vi "ConvertPrefStrings.vi"(6 "Comma?":bool, 8 "String In":string, 11 "Settings":T1={"Name of test"="", "Date"=timestamp(0 s since 1904-01-01), "Location"="Home", "Template"="Simple", "Soundcard"="OCTA-CAPTURE", "resolution"=32, "Sampling rate"=48000, "Ch1 Gain "=25.0, "Ch2 Gain"=10.0, "Sample time (s)"=0.3, "Pre-trigger (s)"=0.001, "Hammer Threshold"=10.0, "Positions"=12, "Taps/Position"=5, "Set Names"="H,V", "Freq resolution"=1.0, "Hammer cutoff"=0.025, "Mic cutoff"=0.25, "Double bounce "=10.0, "Hammer Cal"=10.0, "dB Offset"=0.0, "Accel Cal"=10.0, "Vibrometer Cal"=0.0, "Mic Cal"=0.0, "Output"=2, "Voltage Cal"=0.01, "Vibrometer Port"="ASRL27::INSTR", "Range"=4, "High Pass"=2, "Bandwidth"=4, "X Range"=[], "Y Range"=[], "dB Spread"=0.0, "Trigger"=0, "Ch_1"=25, "Ch_2"=25, "flip?"=FALSE, "60Hz"=FALSE, "Time offset"=0.0, "Piezo Cal"=1.0, "Default Notes"=""} {"Ch_2" min=1 step=1; "Ch_1" min=1 max=100 step=1; "Trigger" items=["Hammer (force)", "Self-tap", "Spacebar"]; "Bandwidth" items=["1 kHz"=1, "5 kHz"=5, "10 kHz"=10, "25 kHz"=25, "50 kHz"=50, "100 kHz"=100]; "High Pass" items=["Off", "13 Hz", "104 Hz"]; "Range" items=["10 mm/s"=1, "20 mm/s"=2, "50 mm/s"=5, "100 mm/s"=10, "200 mm/s"=20, "500 mm/s"=50, "1 m/s"=100, "2 m/s"=200]; "Output" items=["Accelerometer", "Speed (from acceleration)", "Microphone", "Vibrometer", "Piezo"]; "Voltage Cal" format="%#_13g"; "Ch2 Gain" format="%#_13g"; "Ch1 Gain" format="%#_13g"; "Double bounce" min=0.0; "Mic cutoff" min=0.0 format="%#_4g"; "Hammer cutoff" min=0.0 format="%#_4g"; "Freq resolution" min=0.0; "Pre-trigger (s)" format="%#_13g"; "Date" format="%<%H:%M\n%d/%m/%y>T"; "resolution" items=["16 bit"=16, "24 bit"=24, "32 bit"=32]; "Sampling rate" items=["22050 samp/s"=22050, "44100 samp/s"=44100, "48000 samp/s"=48000]}) -> (0 "Settings":T1={"Name of test"="", "Date"=timestamp(0 s since 1904-01-01), "Location"="", "Template"="", "Soundcard"="", "resolution"=32, "Sampling rate"=48000, "Ch1 Gain "=25.0, "Ch2 Gain"=10.0, "Sample time (s)"=0.3, "Pre-trigger (s)"=0.01, "Hammer Threshold"=10.0, "Positions"=12, "Taps/Position"=5, "Set Names"="", "Freq resolution"=10.0, "Hammer cutoff"=0.0, "Mic cutoff"=0.0, "Double bounce "=0.0, "Hammer Cal"=10.0, "dB Offset"=0.0, "Accel Cal"=10.0, "Vibrometer Cal"=0.0, "Mic Cal"=0.0, "Output"=2, "Voltage Cal"=0.01, "Vibrometer Port"="ASRL27::INSTR", "Range"=4, "High Pass"=2, "Bandwidth"=4, "X Range"=[], "Y Range"=[], "dB Spread"=0.0, "Trigger"=0, "Ch_1"=25, "Ch_2"=25, "flip?"=FALSE, "60Hz"=FALSE, "Time offset"=0.0, "Piezo Cal"=1.0, "Default Notes"=""} {"Ch_2" min=1 step=1; "Ch_1" min=1 max=100 step=1; "Trigger" items=["Hammer (force)", "Self-tap", "Spacebar"]; "Bandwidth" items=["1 kHz"=1, "5 kHz"=5, "10 kHz"=10, "25 kHz"=25, "50 kHz"=50, "100 kHz"=100]; "High Pass" items=["Off", "13 Hz", "104 Hz"]; "Range" items=["10 mm/s"=1, "20 mm/s"=2, "50 mm/s"=5, "100 mm/s"=10, "200 mm/s"=20, "500 mm/s"=50, "1 m/s"=100, "2 m/s"=200]; "Output" items=["Accelerometer", "Speed (from acceleration)", "Microphone", "Vibrometer", "Piezo"]; "Voltage Cal" format="%#_13g"; "Ch2 Gain" format="%#_13g"; "Ch1 Gain" format="%#_13g"; "Double bounce" min=0.0; "Mic cutoff" min=0.0 format="%#_4g"; "Hammer cutoff" min=0.0 format="%#_4g"; "Freq resolution" min=0.0; "Pre-trigger (s)" format="%#_13g"; "Date" format="%<%H:%M\n%d/%m/%y>T"; "resolution" items=["16 bit"=16, "24 bit"=24, "32 bit"=32]; "Sampling rate" items=["22050 samp/s"=22050, "44100 samp/s"=44100, "48000 samp/s"=48000]}, 3 "String Out":string)   [LabVIEW 2022 SP3]
uses:
  PreferencesControl.ctl
  <vilib>/Utility/error.llb/Trim Whitespace One-Sided.vi
  Mic/Mic_Global.vi
panel:
  # "Hz"
  # "dB"
  # "dB"
  # "sec"
  # "sec"
  # "mV/Pa"
  # "mV/m/s2"
  # "mV/mm/s"
  # "V/N"
  # "sec"
  # "sec"
  # "mV/N"
  # "a.u."
  # "a.u."
  # "sec"
  # "Hz"
  # "dB"
  # "dB"
  # "sec"
  # "sec"
  # "mV/Pa"
  # "mV/m/s2"
  # "mV/mm/s"
  # "V/N"
  # "sec"
  # "sec"
  # "mV/N"
  # "a.u."
  # "a.u."
  # "sec"
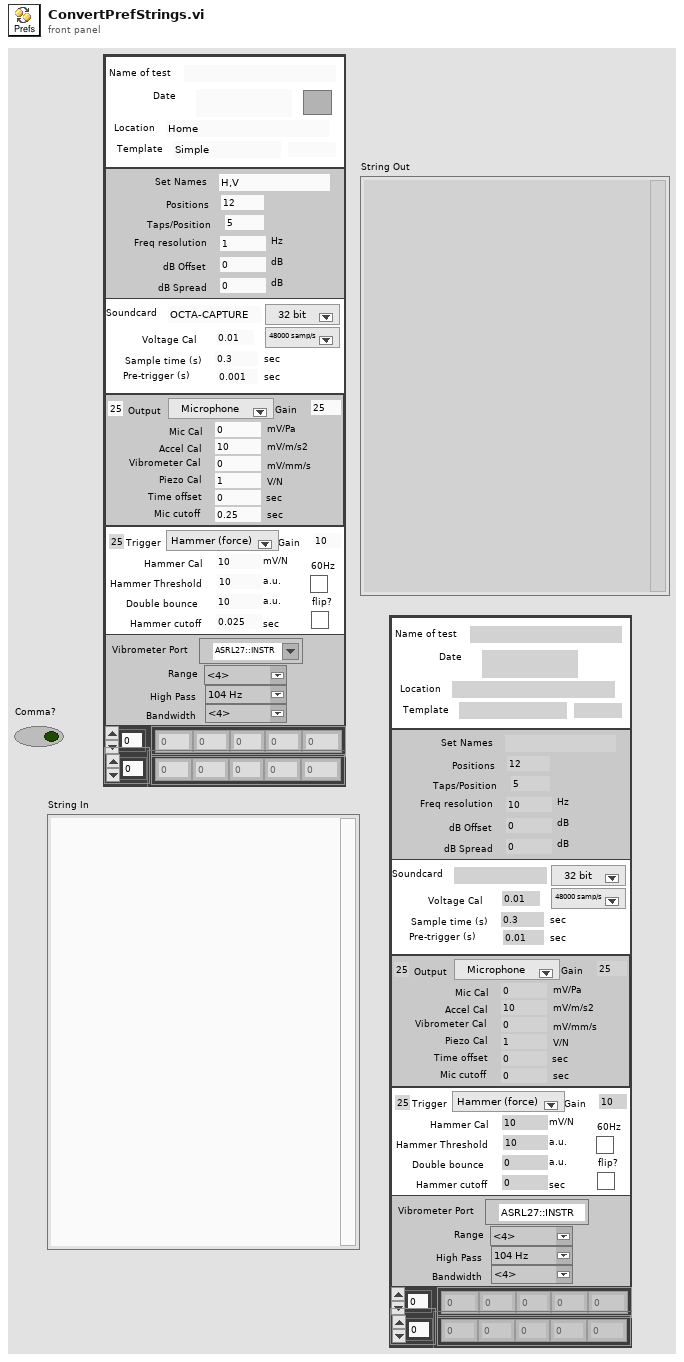
[diagram p1: front panel]
types:
  T1 = typedef "PreferencesControl.ctl" = cluster{"Name of test":string, "Date":timestamp, "Location":string, "Template":string, "Soundcard":string, "resolution":u16, "Sampling rate":u16, "Ch1 Gain ":dbl, "Ch2 Gain":dbl, "Sample time (s)":dbl, "Pre-trigger (s)":dbl, "Hammer Threshold":dbl, "Positions":i16, "Taps/Position":i16, "Set Names":string, "Freq resolution":dbl, "Hammer cutoff":dbl, "Mic cutoff":dbl, "Double bounce ":dbl, "Hammer Cal":dbl, "dB Offset":dbl, "Accel Cal":dbl, "Vibrometer Cal":dbl, "Mic Cal":dbl, "Output":u16, "Voltage Cal":dbl, "Vibrometer Port":refnum<visa-resource-name>, "Range":u16, "High Pass":u16, "Bandwidth":u16, "X Range":cluster{"Minimum":dbl, "Maximum":dbl, "Increment":dbl, "Minor Increment":dbl, "Start":dbl}[], "Y Range":cluster{"Minimum":dbl, "Maximum":dbl, "Increment":dbl, "Minor Increment":dbl, "Start":dbl}[], "dB Spread":dbl, "Trigger":u16, "Ch_1":u8, "Ch_2":u8, "flip?":bool, "60Hz":bool, "Time offset":dbl, "Piezo Cal":dbl, "Default Notes":string}
  T2 = typedef "LVStringsAndValuesArrayTypeDef_U16.ctl" = cluster{"String":string, "Value":u16}[]
  T3 = cluster{"Minimum":dbl, "Maximum":dbl, "Increment":dbl, "Minor Increment":dbl, "Start":dbl}[]
  T4 = cluster{"[0]":dbl, "[1]":dbl, "[2]":dbl, "[3]":dbl, "[4]":dbl}
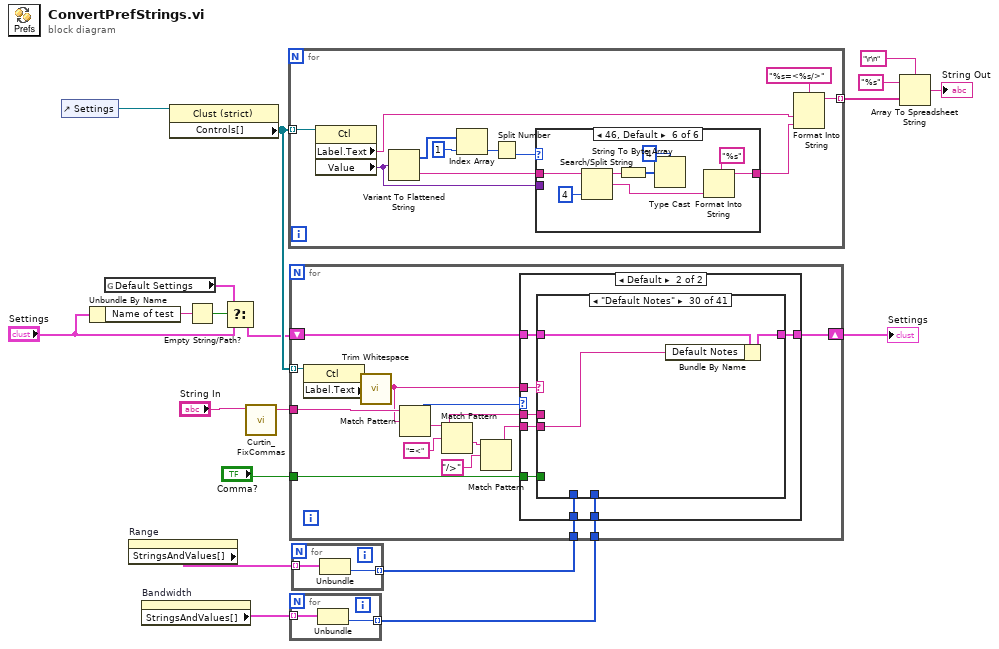
[diagram p0: block diagram]
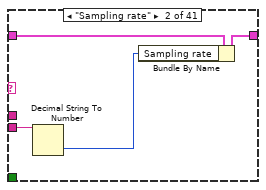
[diagram p4: hidden frame]
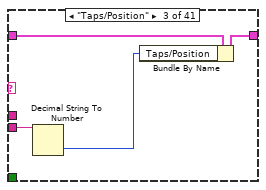
[diagram p5: hidden frame]
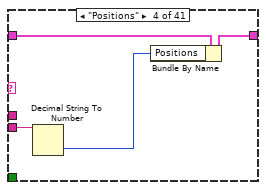
[diagram p6: hidden frame]
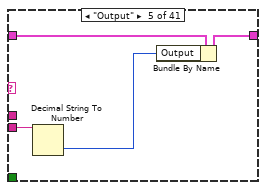
[diagram p7: hidden frame]
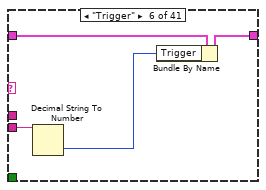
[diagram p8: hidden frame]
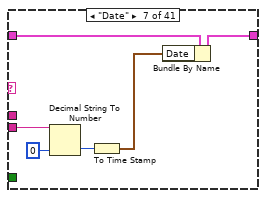
[diagram p9: hidden frame]
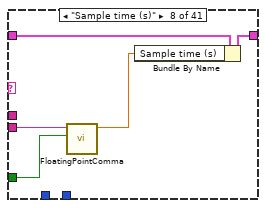
[diagram p10: hidden frame]
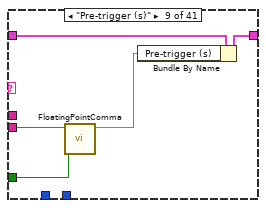
[diagram p11: hidden frame]
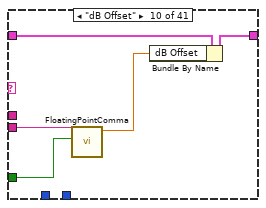
[diagram p12: hidden frame]
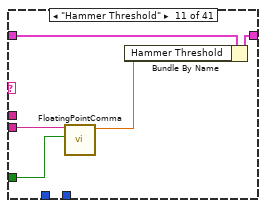
[diagram p13: hidden frame]
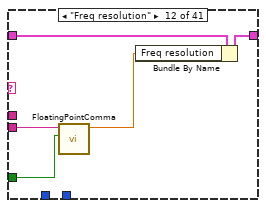
[diagram p14: hidden frame]
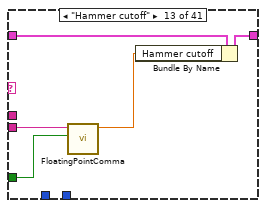
[diagram p15: hidden frame]
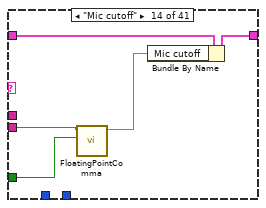
[diagram p16: hidden frame]
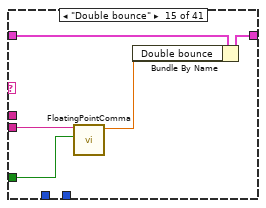
[diagram p17: hidden frame]
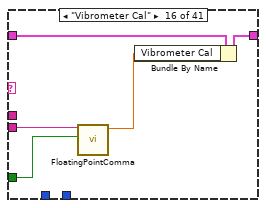
[diagram p18: hidden frame]
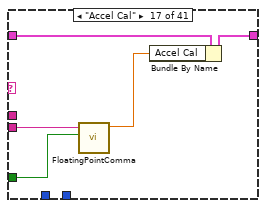
[diagram p19: hidden frame]
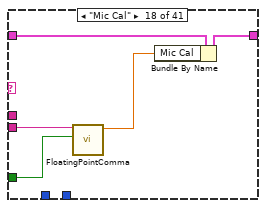
[diagram p20: hidden frame]
diagram:
  n1 = control-ref of="Settings"() -> (w13:refnum<vi>)
  n2 = Unbundle By Name("Settings") -> ("Name of test"=w12:string)
  n3 = global read "Mic_Global.vi" "Default Settings"() -> (w8:T1)
  n4 = property on="Range" class="Ring (strict)"() -> ("StringsAndValues[]"=w5:T2)  [unwired: 2 in, 2 out]
  n5 = property on="Bandwidth" class="Ring (strict)"() -> ("StringsAndValues[]"=w2:T2)  [unwired: 2 in, 2 out]
  n6 = property class="Clust (strict)"(reference=w13) -> ("Controls[]"=w15:refnum<vi>[])  [unwired: 1 in, 2 out]
  n7 = Empty String/Path?(string/path=w12) -> (empty?=w11:bool)
  n8 = Select(t=w8, s=w11, f="Settings") -> (s? t:f=w9:T1)
  n9 = call "Curtin_FixCommas.vi"("String In"="String In") -> ("String In 2"=w6:string)  [unwired: 10 in]
  n10 = for {
    tunnel: w15 -> [w30] mode=indexing
    tunnel: [w28] -> w19 mode=indexing
    n11 = property class="Ctl"(reference=w30) -> ("Label.Text"=w21:string, "Value"=w22:variant)  [unwired: 1 in, 2 out]
    n12 = Variant To Flattened String(Variant=w22) -> (data string=w23:string, 1:w27:i16[])
    n13 = Index Array(array=w27, index=1) -> (element=w26:i16)
    n14 = Split Number(x=w26) -> (lo(x)=w20:u8)  [unwired: 1 out]
    n15 = case shown="46, Default" w20 {
      tunnel: w22 -> [w34 w38 w44 w49 w55 _]
      tunnel: [w31 w35 w40 w45 w51 w62] -> w24
      tunnel: w23 -> [_ _ _ _ _ w65]
      frame 1..8 {
        n16 = Variant To Data(type=i64 0, Variant=w34) -> (data=w32:i64)  [unwired: 1 in, 1 out]
        n17 = Number To Decimal String(number=w32) -> (decimal integer string=w31:string)  [unwired: 1 in]
      }
      frame 9..13 {
        n18 = Variant To Data(type=ext 0.0, Variant=w38) -> (data=w36:ext)  [unwired: 1 in, 1 out]
        n19 = Number To Fractional String(number=w36) -> (F-format string=w35:string)  [unwired: 3 in]
      }
      frame 31, 33 {
        n20 = Variant To Data(type=FALSE, Variant=w44) -> (data=w42:bool)  [unwired: 1 in, 1 out]
        n21 = Select(t="true", s=w42, f="false") -> (s? t:f=w40:string)
      }
      frame 84 {
        n22 = Variant To Data(type=timestamp(0 s since 1904-01-01), Variant=w49) -> (data=w47:timestamp)  [unwired: 1 in, 1 out]
        n23 = To Unsigned Quad Integer(1:w47) -> (0:w46:u64)
        n24 = Number To Decimal String(number=w46) -> (decimal integer string=w45:string)  [unwired: 1 in]
      }
      frame 64 {
        n25 = Variant To Data(type=T3 [] ("X Range"), Variant=w55) -> (data=w53:T3)  [unwired: 1 in, 1 out]
        n26 = for {
          tunnel: w53 -> [w57] mode=indexing
          tunnel: [w56] -> w52 mode=indexing
          n27 = Cluster To Array(cluster=w57) -> (array=w56:dbl[])
        }
        n28 = Array To Spreadsheet String(array=w52, 3:"%e" ("format string")) -> (spreadsheet string=w51:string)  [unwired: 1 in]
      }
      frame 46, Default {
        n29 = Search/Split String(string=w65, offset (0)=4) -> (substring before match=w60:string, match + rest of string=w63:string)  [unwired: 1 in, 1 out]
        n30 = String To Byte Array(string=w60) -> (unsigned byte array=w59:u8[])
        n31 = Type Cast(type=4 ("offset (0)"), x=w59) -> ()  [unwired: 1 out]
        n32 = Format Into String(format string="%s", w63) -> (resulting string=w62:string)  [unwired: 2 in, 1 out]
      }
    }
    n33 = Format Into String(format string="%s=<%s/>", w21, w24) -> (resulting string=w28:string)  [unwired: 2 in, 1 out]
  }
  n34 = for {
    tunnel: w2 -> [w67] mode=indexing
    tunnel: [w66] -> w3 mode=indexing
    n35 = Unbundle(w67) -> ("Value"=w66:u16)  [unwired: 1 out]
  }
  n36 = for {
    tunnel: w5 -> [w69] mode=indexing
    tunnel: [w68] -> w4 mode=indexing
    n37 = Unbundle(w69) -> ("Value"=w68:u16)  [unwired: 1 out]
  }
  n38 = for {
    tunnel: w6 -> [w75]
    tunnel: w15 -> [w81] mode=indexing
    shift-right: [w79] -> w14
    shift-left: w9 -> [w80]
    tunnel: w4 -> [w72]
    tunnel: w3 -> [w71]
    tunnel: "Comma?" -> [w70]
    n39 = property class="Ctl"(reference=w81) -> ("Label.Text"=w74:string)  [unwired: 1 in, 2 out]
    n40 = call <vilib>:"Trim Whitespace.vi"("string"=w74) -> ("trimmed string"=w73:string)  [unwired: 1 in]
    n41 = Match Pattern(string=w75, regular expression=w73) -> (after substring=w76:string, offset past match=w77:i32)  [unwired: 1 in, 2 out]
    n42 = Match Pattern(string=w76, regular expression="=<" ("format string")) -> (after substring=w82:string)  [unwired: 1 in, 3 out]
    n43 = Match Pattern(string=w82, regular expression="/>" ("format string")) -> (before substring=w78:string)  [unwired: 1 in, 3 out]
    n44 = case shown="Default" w77 {
      tunnel: w80 -> [w85 w93]
      tunnel: [w85 w92] -> w79
      tunnel: w73 -> [_ w91]
      tunnel: w78 -> [_ w90]
      tunnel: w76 -> [_ w89]
      tunnel: w72 -> [_ w88]
      tunnel: w71 -> [_ w87]
      tunnel: w70 -> [_ w86]
      frame -1 {
      }
      frame Default {
        n45 = case shown="\"Default Notes\"" w91 {
          tunnel: w93 -> [w94 w98 w102 w106 w110 w114 w120 w125 w130 w135 w140 w145 w150 w155 w160 w165 w170 w175 w180 w184 w187 w190 w193 w196 w199 w204 w209 w214 w217 w220 w229 w233 w242 w250 w260 w267 w271 w275 w280 w285 w290]
          tunnel: [w94 w97 w101 w105 w109 w113 w119 w124 w129 w134 w139 w144 w149 w154 w159 w164 w169 w174 w179 w183 w186 w189 w192 w195 w198 w203 w208 w213 w216 w219 w228 w232 w241 w249 w259 w266 w270 w274 w279 w284 w289] -> w92
          tunnel: w90 -> [_ w96 w100 w104 w108 w112 w118 w123 w128 w133 w138 w143 w148 w153 w158 w163 w168 w173 w178 w182 w185 w188 w191 w194 w197 w202 w207 w211 w215 w218 w222 w231 w240 w245 w255 w265 w269 w273 w277 w282 w288]
          tunnel: w89 -> [_ _ _ _ _ _ _ _ _ _ _ _ _ _ _ _ _ _ _ _ _ _ _ _ _ _ _ _ _ _ _ _ _ _ _ _ _ _ _ _ _]
          tunnel: w88 -> [_ _ _ _ _ _ _ _ _ _ _ _ _ _ _ _ _ _ _ _ _ _ _ _ _ _ _ _ _ _ w221 _ _ _ _ _ _ _ _ _ _]
          tunnel: w87 -> [_ _ _ _ _ _ _ _ _ _ _ _ _ _ _ _ _ _ _ _ _ _ _ _ _ _ _ _ _ _ _ _ w236 _ _ _ _ _ _ _ _]
          tunnel: w86 -> [_ _ _ _ _ _ _ w121 w127 w132 w137 w142 w147 w152 w157 w162 w167 w172 w177 _ _ _ _ _ _ w201 w206 w212 _ _ _ _ _ w244 w254 w264 _ _ _ _ w287]
          frame Default {
          }
          frame "Sampling rate" {
            n46 = Decimal String To Number(string=w96) -> (number=w95:i32)  [unwired: 2 in, 1 out]
            n47 = Bundle By Name(cluster=w98, "Sampling rate"=w95) -> (w97:T1)
          }
          frame "Taps/Position" {
            n48 = Decimal String To Number(string=w100) -> (number=w99:i32)  [unwired: 2 in, 1 out]
            n49 = Bundle By Name(cluster=w102, "Taps/Position"=w99) -> (w101:T1)
          }
          frame "Positions" {
            n50 = Decimal String To Number(string=w104) -> (number=w103:i32)  [unwired: 2 in, 1 out]
            n51 = Bundle By Name(cluster=w106, "Positions"=w103) -> (w105:T1)
          }
          frame "Output" {
            n52 = Decimal String To Number(string=w108) -> (number=w107:i32)  [unwired: 2 in, 1 out]
            n53 = Bundle By Name(cluster=w110, "Output"=w107) -> (w109:T1)
          }
          frame "Trigger" {
            n54 = Decimal String To Number(string=w112) -> (number=w111:i32)  [unwired: 2 in, 1 out]
            n55 = Bundle By Name(cluster=w114, "Trigger"=w111) -> (w113:T1)
          }
          frame "Date" {
            n56 = Decimal String To Number(string=w118, default (0L)=u64 0 ("default (0 I32)")) -> (number=w117:u64)  [unwired: 1 in, 1 out]
            n57 = To Time Stamp(1:w117) -> (0:w116:timestamp)
            n58 = Bundle By Name(cluster=w120, "Date"=w116) -> (w119:T1)
          }
          frame "Sample time (s)" {
            n59 = call "FloatingPointComma.vi"("Comma?"=w121, "String In"=w123) -> ("Numeric"=w122:dbl)  [unwired: 8 in, 1 out]
            n60 = Bundle By Name(cluster=w125, "Sample time (s)"=w122) -> (w124:T1)
          }
          frame "Pre-trigger (s)" {
            n61 = call "FloatingPointComma.vi"("Comma?"=w127, "String In"=w128) -> ("Numeric"=w126:dbl)  [unwired: 8 in, 1 out]
            n62 = Bundle By Name(cluster=w130, "Pre-trigger (s)"=w126) -> (w129:T1)
          }
          frame "dB Offset" {
            n63 = call "FloatingPointComma.vi"("Comma?"=w132, "String In"=w133) -> ("Numeric"=w131:dbl)  [unwired: 8 in, 1 out]
            n64 = Bundle By Name(cluster=w135, "dB Offset"=w131) -> (w134:T1)
          }
          frame "Hammer Threshold" {
            n65 = call "FloatingPointComma.vi"("Comma?"=w137, "String In"=w138) -> ("Numeric"=w136:dbl)  [unwired: 8 in, 1 out]
            n66 = Bundle By Name(cluster=w140, "Hammer Threshold"=w136) -> (w139:T1)
          }
          frame "Freq resolution" {
            n67 = call "FloatingPointComma.vi"("Comma?"=w142, "String In"=w143) -> ("Numeric"=w141:dbl)  [unwired: 8 in, 1 out]
            n68 = Bundle By Name(cluster=w145, "Freq resolution"=w141) -> (w144:T1)
          }
          frame "Hammer cutoff" {
            n69 = call "FloatingPointComma.vi"("Comma?"=w147, "String In"=w148) -> ("Numeric"=w146:dbl)  [unwired: 8 in, 1 out]
            n70 = Bundle By Name(cluster=w150, "Hammer cutoff"=w146) -> (w149:T1)
          }
          frame "Mic cutoff" {
            n71 = call "FloatingPointComma.vi"("Comma?"=w152, "String In"=w153) -> ("Numeric"=w151:dbl)  [unwired: 8 in, 1 out]
            n72 = Bundle By Name(cluster=w155, "Mic cutoff"=w151) -> (w154:T1)
          }
          frame "Double bounce" {
            n73 = call "FloatingPointComma.vi"("Comma?"=w157, "String In"=w158) -> ("Numeric"=w156:dbl)  [unwired: 8 in, 1 out]
            n74 = Bundle By Name(cluster=w160, "Double bounce"=w156) -> (w159:T1)
          }
          frame "Vibrometer Cal" {
            n75 = call "FloatingPointComma.vi"("Comma?"=w162, "String In"=w163) -> ("Numeric"=w161:dbl)  [unwired: 8 in, 1 out]
            n76 = Bundle By Name(cluster=w165, "Vibrometer Cal"=w161) -> (w164:T1)
          }
          frame "Accel Cal" {
            n77 = call "FloatingPointComma.vi"("Comma?"=w167, "String In"=w168) -> ("Numeric"=w166:dbl)  [unwired: 8 in, 1 out]
            n78 = Bundle By Name(cluster=w170, "Accel Cal"=w166) -> (w169:T1)
          }
          frame "Mic Cal" {
            n79 = call "FloatingPointComma.vi"("Comma?"=w172, "String In"=w173) -> ("Numeric"=w171:dbl)  [unwired: 8 in, 1 out]
            n80 = Bundle By Name(cluster=w175, "Mic Cal"=w171) -> (w174:T1)
          }
          frame "Hammer Cal" {
            n81 = call "FloatingPointComma.vi"("Comma?"=w177, "String In"=w178) -> ("Numeric"=w176:dbl)  [unwired: 8 in, 1 out]
            n82 = Bundle By Name(cluster=w180, "Hammer Cal"=w176) -> (w179:T1)
          }
          frame "resolution" {
            n83 = Decimal String To Number(string=w182) -> (number=w181:i32)  [unwired: 2 in, 1 out]
            n84 = Bundle By Name(cluster=w184, "resolution"=w181) -> (w183:T1)
          }
          frame "Soundcard" {
            n85 = Bundle By Name(cluster=w187, "Soundcard"=w185) -> (w186:T1)
          }
          frame "Name of test" {
            n86 = Bundle By Name(cluster=w190, "Name of test"=w188) -> (w189:T1)
          }
          frame "Set Names" {
            n87 = Bundle By Name(cluster=w193, "Set Names"=w191) -> (w192:T1)
          }
          frame "Location" {
            n88 = Bundle By Name(cluster=w196, "Location"=w194) -> (w195:T1)
          }
          frame "Default Template" {
            n89 = Bundle By Name(cluster=w199, "Template"=w197) -> (w198:T1)
          }
          frame "Ch1 Gain" {
            n90 = call "FloatingPointComma.vi"("Comma?"=w201, "String In"=w202) -> ("Numeric"=w200:dbl)  [unwired: 8 in, 1 out]
            n91 = Bundle By Name(cluster=w204, "Ch1 Gain"=w200) -> (w203:T1)
          }
          frame "Ch2 Gain" {
            n92 = call "FloatingPointComma.vi"("Comma?"=w206, "String In"=w207) -> ("Numeric"=w205:dbl)  [unwired: 8 in, 1 out]
            n93 = Bundle By Name(cluster=w209, "Ch2 Gain"=w205) -> (w208:T1)
          }
          frame "Voltage Cal" {
            n94 = call "FloatingPointComma.vi"("Comma?"=w212, "String In"=w211) -> ("Numeric"=w210:dbl)  [unwired: 8 in, 1 out]
            n95 = Bundle By Name(cluster=w214, "Voltage Cal"=w210) -> (w213:T1)
          }
          frame "Vibrometer Port" {
            n96 = Bundle By Name(cluster=w217, "Vibrometer Port"=w215) -> (w216:T1)
          }
          frame "Default Notes" {
            n97 = Bundle By Name(cluster=w220, "Default Notes"=w218) -> (w219:T1)
          }
          frame "Range" {
            n98 = Decimal String To Number(string=w222) -> (number=w225:i32)  [unwired: 2 in, 1 out]
            n99 = Search 1D Array(1D array=w221, element=w225) -> (index of element=w227:i32)  [unwired: 1 in]
            n100 = Greater Or Equal To 0?(x=w227) -> (x >= 0?=w226:bool)
            n101 = Select(t=w225, s=w226, f=20) -> (s? t:f=w224:i32)
            n102 = Bundle By Name(cluster=w229, "Range"=w224) -> (w228:T1)
          }
          frame "High Pass" {
            n103 = Decimal String To Number(string=w231) -> (number=w230:i32)  [unwired: 2 in, 1 out]
            n104 = Bundle By Name(cluster=w233, "High Pass"=w230) -> (w232:T1)
          }
          frame "Bandwidth" {
            n105 = Decimal String To Number(string=w240) -> (number=w235:i32)  [unwired: 2 in, 1 out]
            n106 = Search 1D Array(1D array=w236, element=w235) -> (index of element=w239:i32)  [unwired: 1 in]
            n107 = Greater Or Equal To 0?(x=w239) -> (x >= 0?=w238:bool)
            n108 = Select(t=w235, s=w238, f=25) -> (s? t:f=w234:i32)
            n109 = Bundle By Name(cluster=w242, "Bandwidth"=w234) -> (w241:T1)
          }
          frame "X Range" {
            n110 = call "FloatingPointComma.vi"("Comma?"=w244, "String In"=w245) -> ("fixed"=w243:string)  [unwired: 8 in, 1 out]
            n111 = Spreadsheet String To Array(format string="%e", spreadsheet string=w243) -> (array=w247:dbl[][])  [unwired: 2 in]
            n112 = for {
              tunnel: w247 -> [w252] mode=indexing
              tunnel: [w251] -> w246 mode=indexing
              n113 = Array To Cluster(array=w252) -> (cluster=w251:T4)
            }
            n114 = Bundle By Name(cluster=w250, "X Range"=w246) -> (w249:T1)
          }
          frame "Y Range" {
            n115 = call "FloatingPointComma.vi"("Comma?"=w254, "String In"=w255) -> ("fixed"=w253:string)  [unwired: 8 in, 1 out]
            n116 = Spreadsheet String To Array(format string="%e", spreadsheet string=w253) -> (array=w257:dbl[][])  [unwired: 2 in]
            n117 = for {
              tunnel: w257 -> [w262] mode=indexing
              tunnel: [w261] -> w256 mode=indexing
              n118 = Array To Cluster(array=w262) -> (cluster=w261:T4)
            }
            n119 = Bundle By Name(cluster=w260, "Y Range"=w256) -> (w259:T1)
          }
          frame "dB Spread" {
            n120 = call "FloatingPointComma.vi"("Comma?"=w264, "String In"=w265) -> ("Numeric"=w263:dbl)  [unwired: 8 in, 1 out]
            n121 = Bundle By Name(cluster=w267, "dB Spread"=w263) -> (w266:T1)
          }
          frame "Ch_1" {
            n122 = Decimal String To Number(string=w269) -> (number=w268:i32)  [unwired: 2 in, 1 out]
            n123 = Bundle By Name(cluster=w271, "Ch_1"=w268) -> (w270:T1)
          }
          frame "Ch_2" {
            n124 = Decimal String To Number(string=w273) -> (number=w272:i32)  [unwired: 2 in, 1 out]
            n125 = Bundle By Name(cluster=w275, "Ch_2"=w272) -> (w274:T1)
          }
          frame "flip?" {
            n126 = Equal?(x="true", y=w277) -> (x = y?=w276:bool)
            n127 = Bundle By Name(cluster=w280, "flip?"=w276) -> (w279:T1)
          }
          frame "60Hz" {
            n128 = Equal?(x="true", y=w282) -> (x = y?=w281:bool)
            n129 = Bundle By Name(cluster=w285, "60Hz"=w281) -> (w284:T1)
          }
          frame "Time offset" {
            n130 = call "FloatingPointComma.vi"("Comma?"=w287, "String In"=w288) -> ("Numeric"=w286:dbl)  [unwired: 8 in, 1 out]
            n131 = Bundle By Name(cluster=w290, "Time offset"=w286) -> (w289:T1)
          }
        }
      }
    }
  }
  "Settings" <- w14
  n132 = Array To Spreadsheet String(delimiter (Tab)="\r\n", array=w19, 3:"%s" ("format string")) -> (spreadsheet string=→"String Out":string)
